vi "Control-CaseFlow.vi"(0 "Camera Device  IN":T1, 1 "Image Device IN":cluster{"Image":T5, "errorImage":errorcluster}, 2 "DAQ Device IN":T3={"DAQ Fs (S/s)"=10000.0, "task"="", "error"={"status"=FALSE, "code"=0, "source"=""}, "Min Value"=-10.0, "Max Value"=10.0}, 3 "Time Control Parameters":cluster{"# samples":u32, "tiempos (ms)":dbl}, 4 "Parametros Maximos":T6, 5 "detla Parametros":T6, 6 "Camara ON?":bool, 7 "Control Parameters":T4={"N Init Avg"=6, "N Avg Best"=3, "% Best to test"=0.95, "% Best to beat"=1.0}, 8 "Control?":bool=TRUE, 9 "Reset Control":bool, 10 "Ajuste?":bool=TRUE, 11 "Calibracion DAQ":T2) -> (13 "Status Text":string, 14 "Camera Device OUT":T1, 15 "Image Device OUT":cluster{"Image":T5, "errorImage":errorcluster}, 16 "DAQ Device OUT":T3={"DAQ Fs (S/s)"=0.0, "task"="", "error"={"status"=FALSE, "code"=0, "source"=""}, "Min Value"=-10.0, "Max Value"=10.0}, 17 "Contraste":dbl, 18 "Waveform":waveform(dbl), 19 "Señal de Control":dbl[](array[numeric]))   [LabVIEW 2010]
uses:
  <vilib>/vision/Image Controls.llb/IMAQ Image.ctl
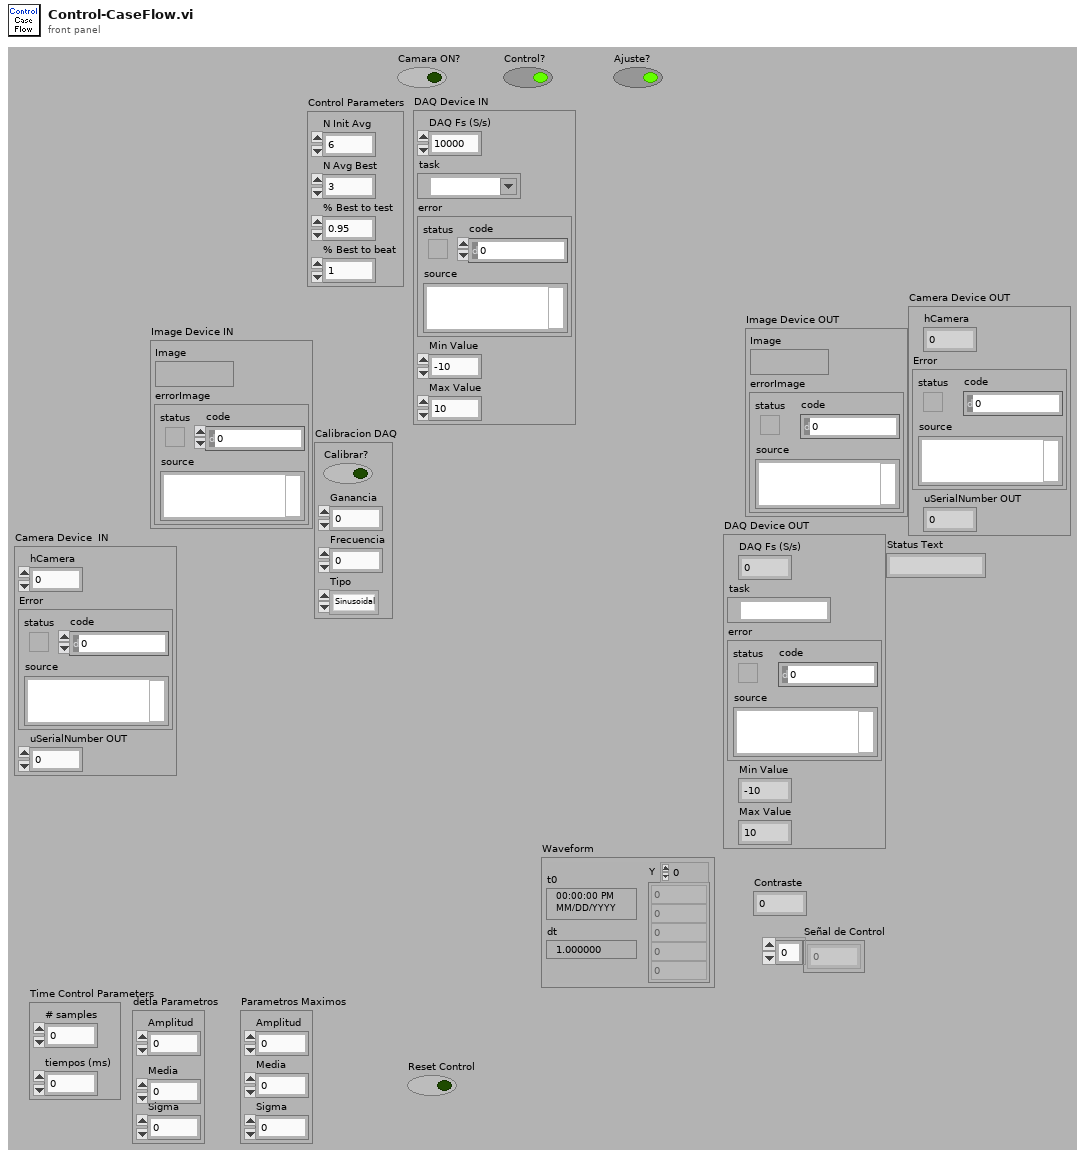
[diagram p1: front panel]
types:
  T1 = cluster{"hCamera":u32, "Error":errorcluster, "uSerialNumber OUT":u32}
  T2 = cluster{"Calibrar?":bool, "Ganancia":dbl, "Frecuencia":dbl, "Tipo":enum16{"Sinusoidal", "Triangular", "Cuadrada"}}
  T3 = cluster{"DAQ Fs (S/s)":dbl, "task":refnum<k21>, "error":errorcluster, "Min Value":dbl, "Max Value":dbl}
  T4 = cluster{"N Init Avg":u32, "N Avg Best":u32, "% Best to test":dbl, "% Best to beat":dbl}
  T5 = typedef "IMAQ Image.ctl" = refnum<image>
  T6 = cluster{"Amplitud":dbl, "Media":dbl, "Sigma":dbl}
  T7 = cluster{"DAQ Limits":cluster{"max":dbl, "min":dbl}, "Control Limits":cluster{"max":dbl, "min":dbl}}
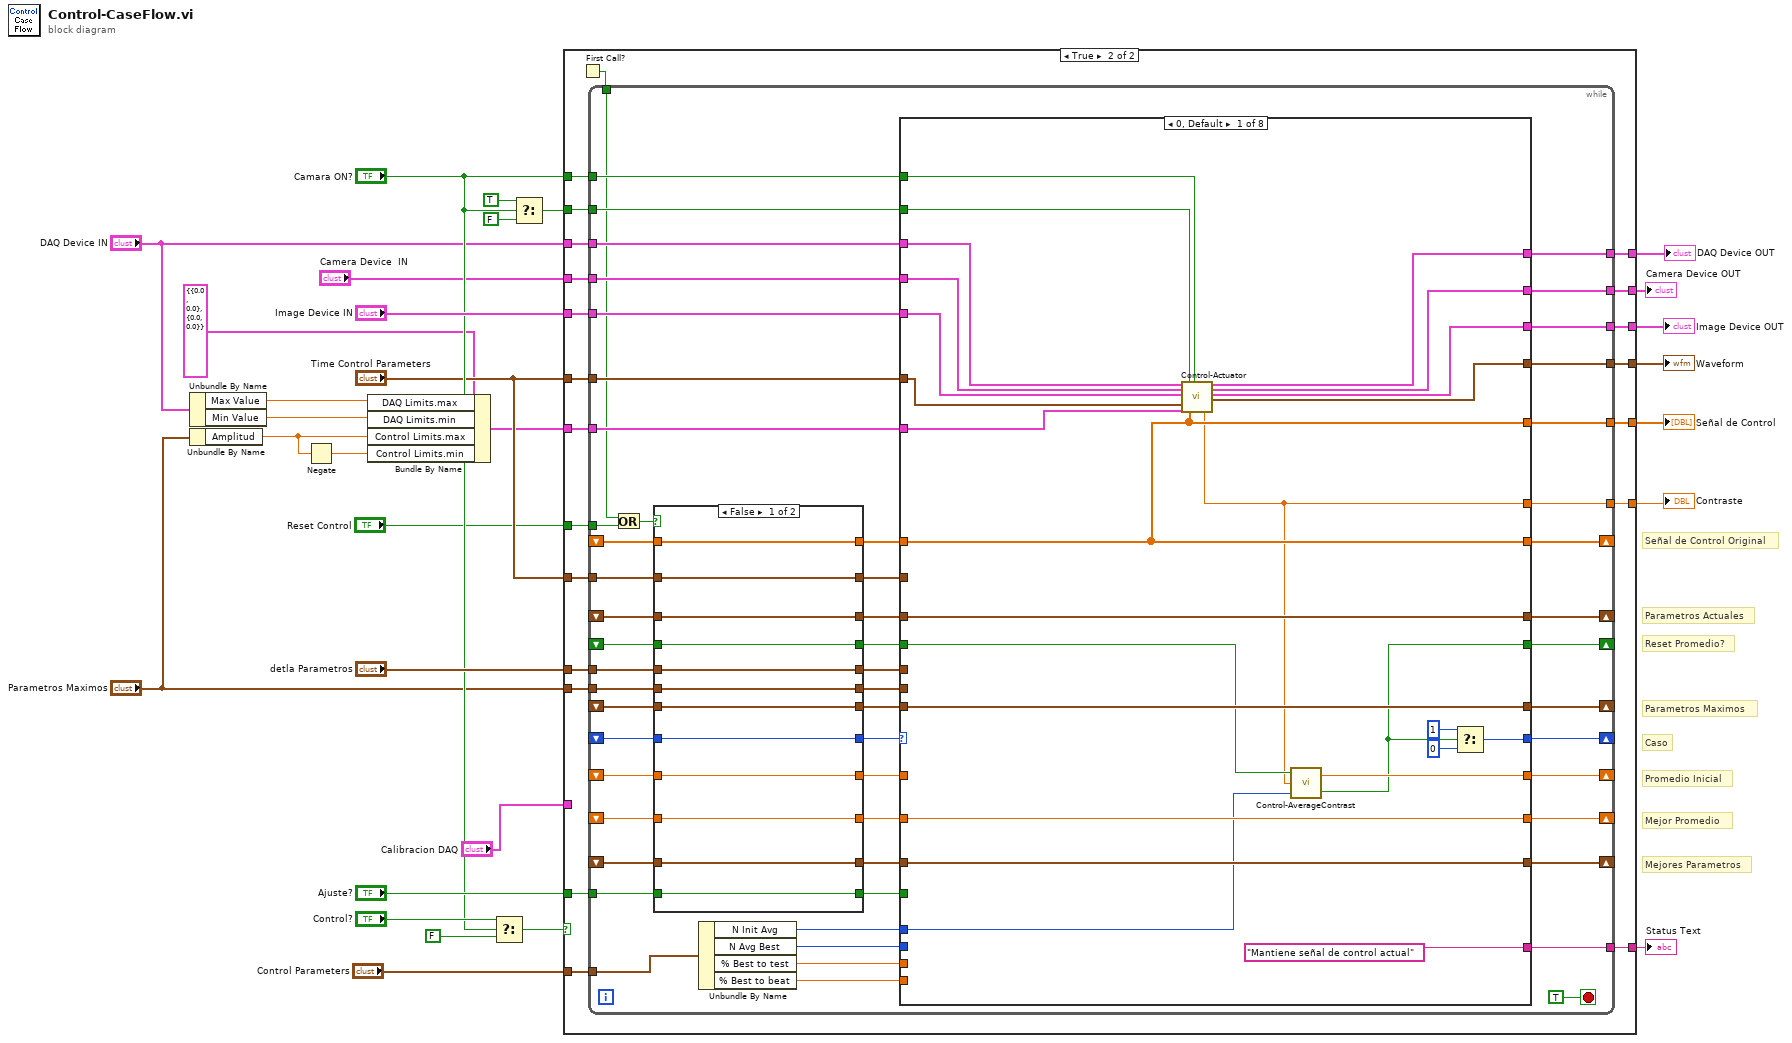
[diagram p0: block diagram]
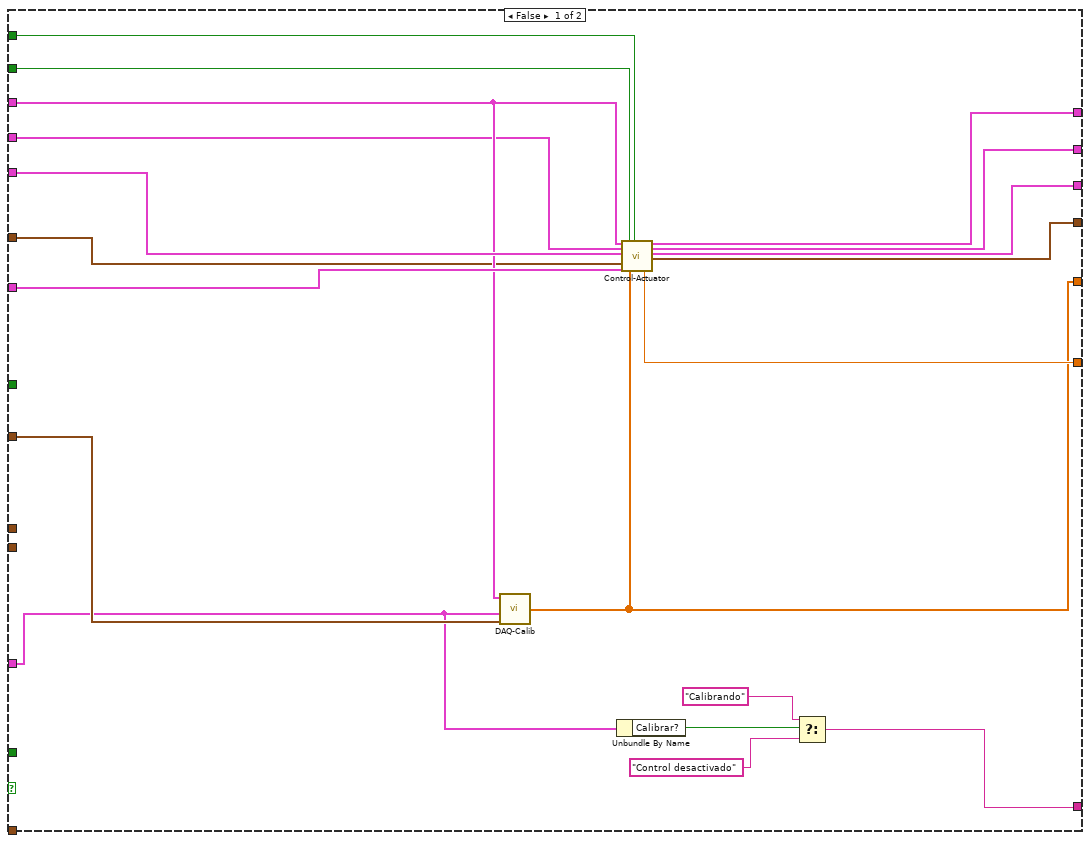
[diagram p2: hidden frame]
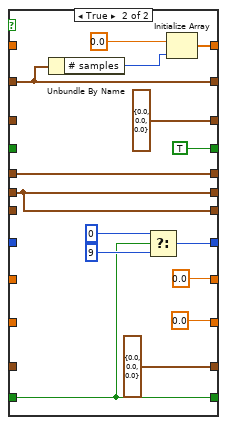
[diagram p3: hidden frame]
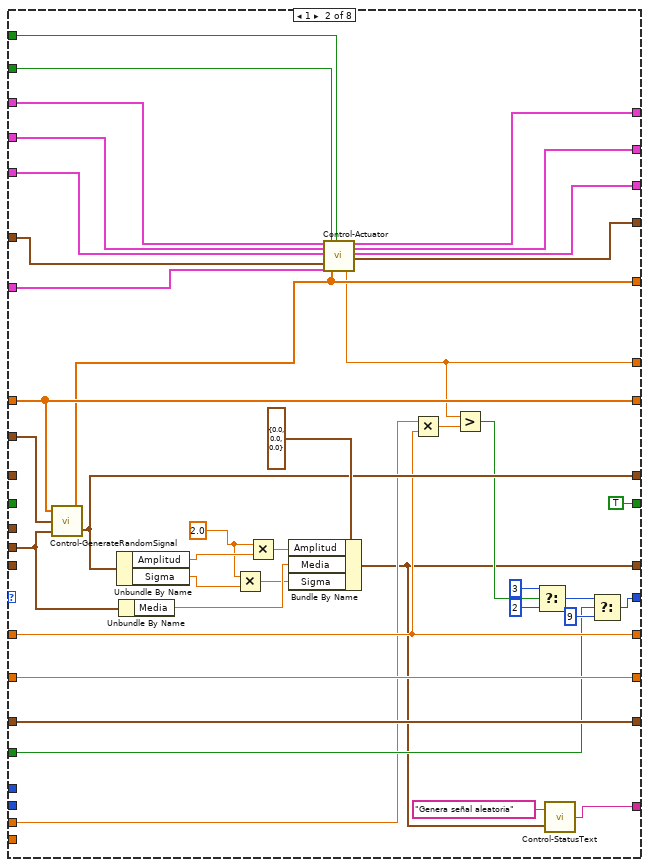
[diagram p4: hidden frame]
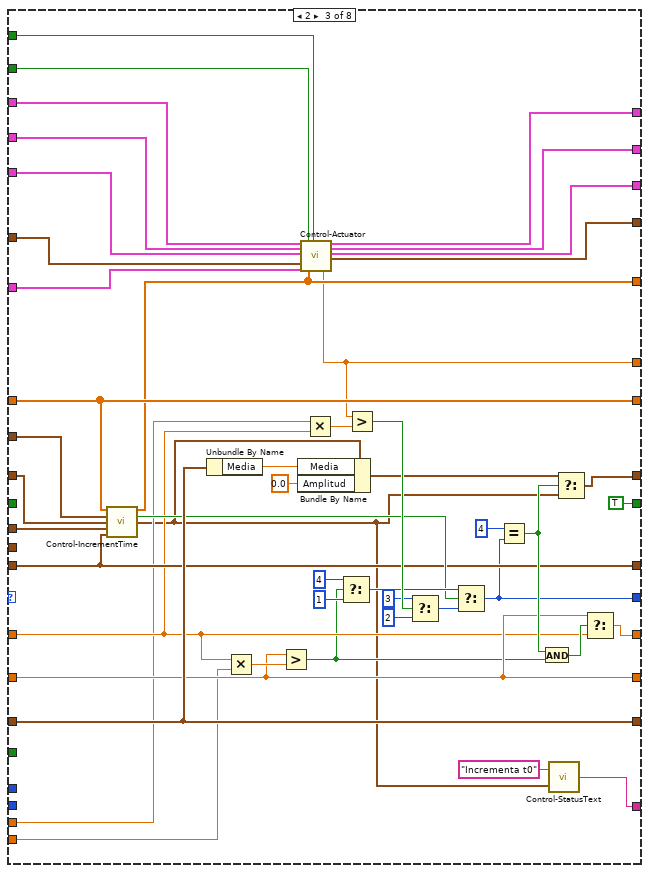
[diagram p5: hidden frame]
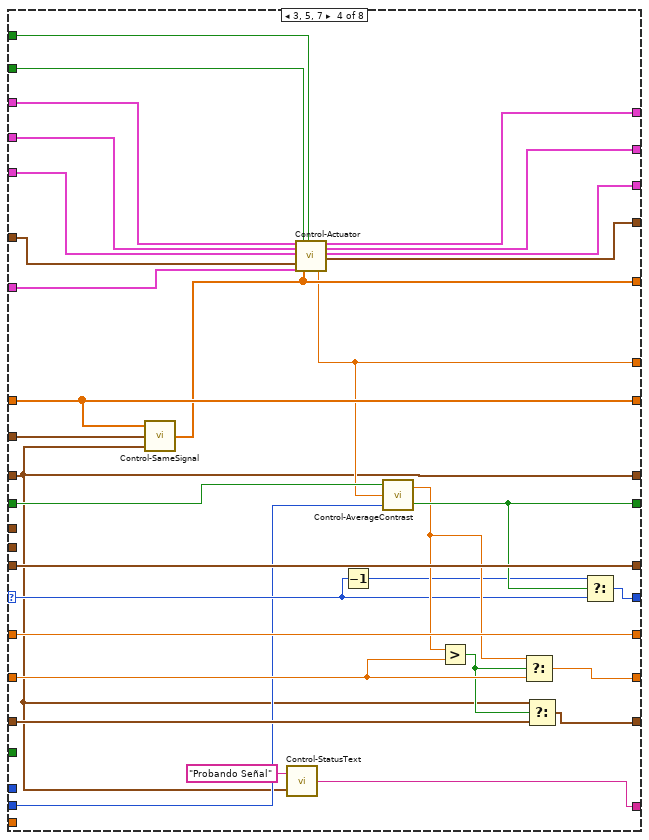
[diagram p6: hidden frame]
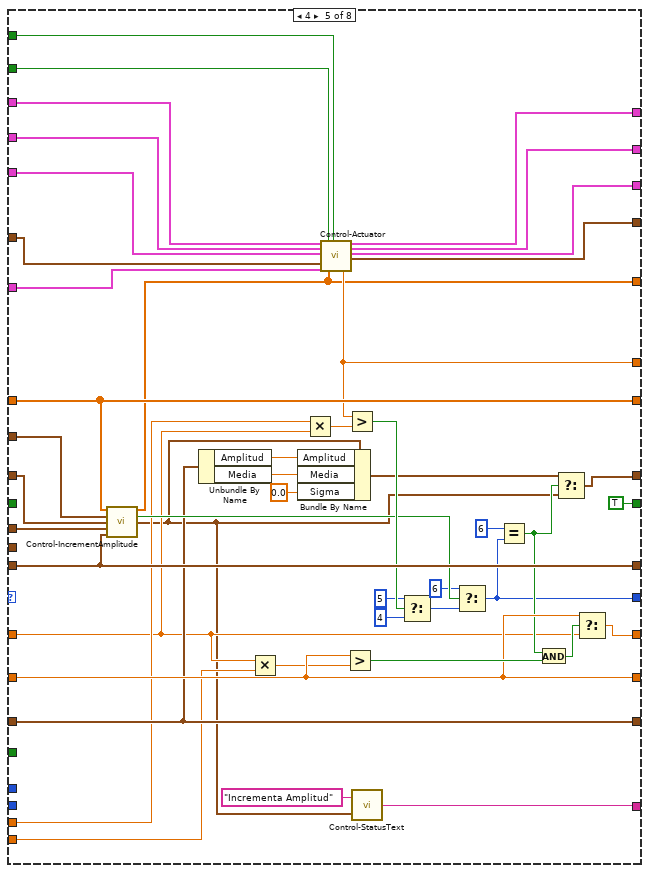
[diagram p7: hidden frame]
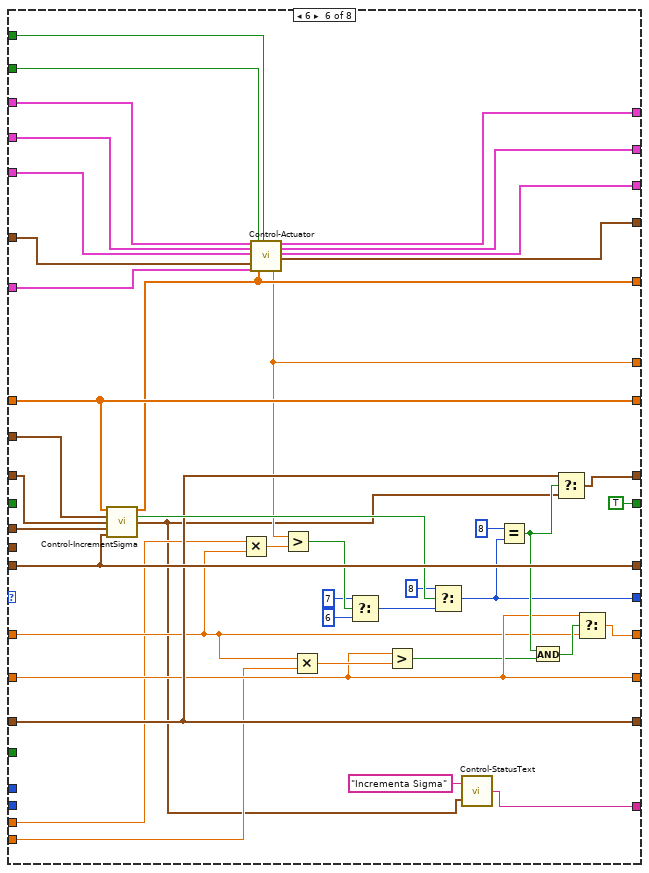
[diagram p8: hidden frame]
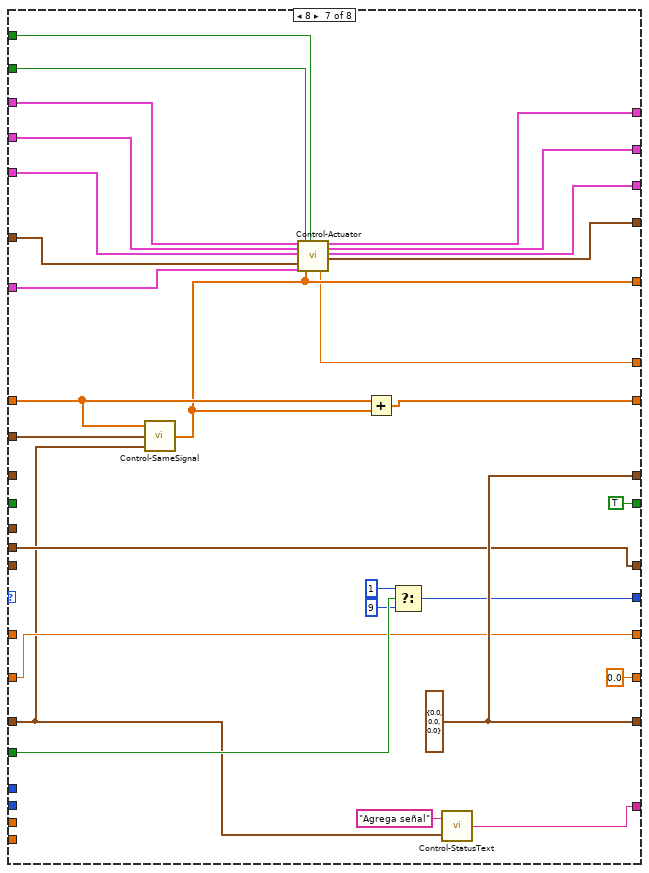
[diagram p9: hidden frame]
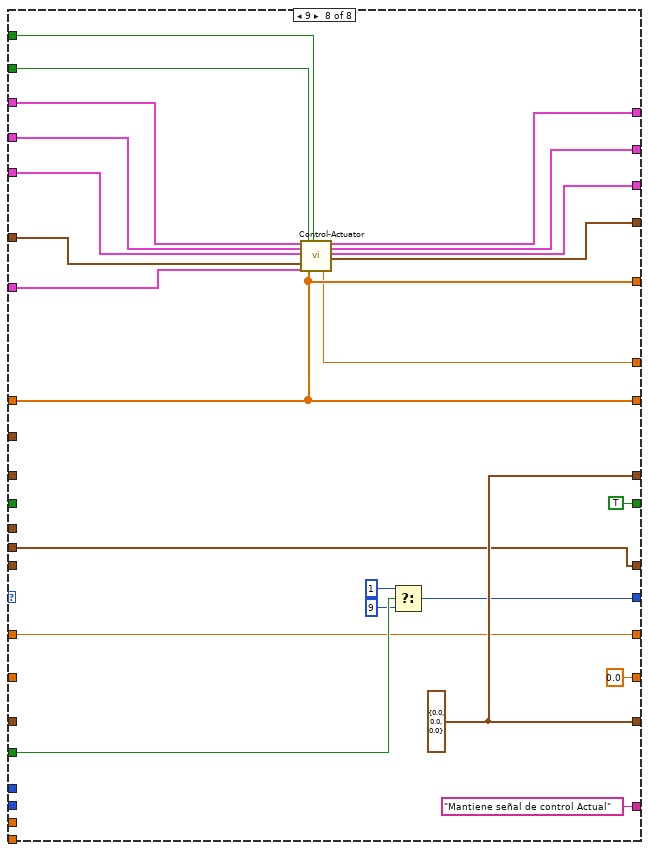
[diagram p10: hidden frame]
diagram:
  # "Reset Promedio?"
  # "Mejores Parametros"
  # "Mejor Promedio"
  # "Señal de Control Original"
  # "Parametros Actuales"
  # "Parametros Maximos"
  # "Caso"
  # "Promedio Inicial"
  n1 = Unbundle By Name("DAQ Device IN") -> ("Max Value"=w10:dbl, "Min Value"=w9:dbl)
  n2 = Unbundle By Name("Parametros Maximos") -> ("Amplitud"=w7:dbl)
  n3 = Negate(x=w7) -> (-x=w8:dbl)
  n4 = Bundle By Name(cluster=T7 {"DAQ Limits"={"max"=0.0, "min"=0.0}, "Control Limits"={"max"=0.0, "min"=0.0}} ("Limites"), "DAQ Limits.max"=w10, "DAQ Limits.min"=w9, "Control Limits.max"=w7, "Control Limits.min"=w8) -> (w11:T7)
  n5 = Select(t="Control?", s="Camara ON?", f=FALSE) -> (s? t:f=w20:bool)
  n6 = Select(t=TRUE, s="Camara ON?", f=FALSE) -> (s? t:f=w23:bool)
  n7 = case shown="True" w20 {
    tunnel: "Time Control Parameters" -> [w37 w70]
    tunnel: "detla Parametros" -> [_ w69]
    tunnel: "Parametros Maximos" -> [_ w68]
    tunnel: "Ajuste?" -> [_ w66]
    tunnel: [w39 w65] -> w28
    tunnel: [w49 w64] -> w27
    tunnel: w11 -> [w48 w63]
    tunnel: "Time Control Parameters" -> [w36 w62]
    tunnel: "Image Device IN" -> [w47 w61]
    tunnel: "Camera Device  IN" -> [w38 w60]
    tunnel: "DAQ Device IN" -> [w40 w59]
    tunnel: w23 -> [w46 w58]
    tunnel: "Camara ON?" -> [w45 w57]
    tunnel: [w44 w56] -> w25
    tunnel: [w43 w55] -> w24
    tunnel: [w42 w54] -> w2
    tunnel: [w41 w53] -> w13
    tunnel: "Reset Control" -> [_ w52]
    tunnel: "Control Parameters" -> [_ w51]
    tunnel: "Calibracion DAQ" -> [w32 _]
    tunnel: [w31 w50] -> w1
    frame False {
      n8 = call "DAQ-Calib.vi"("Time Control Parameters"=w37, "Calibracion DAQ"=w32, "DAQ Device IN"=w40) -> ("Calibration OUT"=w39:dbl[])  [unwired: 1 in]
      n9 = Unbundle By Name(w32) -> ("Calibrar?"=w35:bool)
      n10 = call "Control-Actuator.vi"("DAQ Device IN"=w40, "Camera Device  IN"=w38, "Image Device IN"=w47, "Time Control Parameters"=w36, "Limites"=w48, "DAQ?"=w46, "ControlSignal"=w39, "Streeam?"=w45) -> ("Contraste"=w49:dbl, "DAQ Device OUT"=w41:T3, "Camera Device OUT"=w42:T1, "Image Device OUT"=w43:cluster{"Image":T5, "errorImage":errorcluster}, "Waveform"=w44:waveform(dbl))  [unwired: 7 in]
      n11 = Select(t="Calibrando", s=w35, f="Control desactivado") -> (s? t:f=w31:string)
    }
    frame True {
      n12 = First Call?() -> (First Call?: T/F=w67:bool)
      n13 = while {
        shift-right: [w122] -> _
        shift-left: _ -> [w109]
        tunnel: w70 -> [w101]
        shift-right: [w125] -> _
        shift-left: _ -> [w117]
        shift-right: [w124] -> _
        shift-left: _ -> [w111]
        shift-right: [w123] -> _
        shift-left: _ -> [w115]
        shift-right: [w121] -> _
        shift-left: _ -> [w107]
        tunnel: w69 -> [w98]
        shift-right: [w120] -> _
        shift-left: _ -> [w105]
        shift-right: [w119] -> _
        shift-left: _ -> [w103]
        shift-right: [w118] -> _
        shift-left: _ -> [w113]
        tunnel: w66 -> [w100]
        tunnel: w68 -> [w99]
        tunnel: w67 -> [w79]
        tunnel: [w93] -> w65
        tunnel: [w92] -> w64
        tunnel: w63 -> [w91]
        tunnel: w62 -> [w90]
        tunnel: w61 -> [w89]
        tunnel: w60 -> [w88]
        tunnel: w59 -> [w87]
        tunnel: w58 -> [w86]
        tunnel: w57 -> [w85]
        tunnel: [w84] -> w56
        tunnel: [w83] -> w55
        tunnel: [w82] -> w54
        tunnel: [w81] -> w53
        tunnel: w52 -> [w77]
        tunnel: w51 -> [w76]
        tunnel: [w71] -> w50
        stop <- TRUE stop-if-true
        n14 = Or(x=w79, y=w77) -> (x .or. y?=w78:bool)
        n15 = case shown="False" w78 {
          tunnel: w117 -> [w137 _]
          tunnel: [w137 w152] -> w116
          tunnel: [w136 T6 {"Amplitud"=0.0, "Media"=0.0, "Sigma"=0.0} ("Parametros Iniciales")] -> w114
          tunnel: w115 -> [w136 _]
          tunnel: w113 -> [w135 _]
          tunnel: [w135 TRUE] -> w112
          tunnel: w111 -> [w134 _]
          tunnel: [w134 w141] -> w110
          tunnel: w109 -> [w133 _]
          tunnel: [w133 w142] -> w108
          tunnel: w107 -> [w132 _]
          tunnel: [w132 0.0 ("Contraste Promedio")] -> w106
          tunnel: w105 -> [w131 _]
          tunnel: [w131 0.0 ("Contraste Promedio")] -> w104
          tunnel: w103 -> [w130 _]
          tunnel: [w130 T6 {"Amplitud"=0.0, "Media"=0.0, "Sigma"=0.0} ("Parametros Maximos")] -> w102
          tunnel: w101 -> [w129 w138]
          tunnel: w99 -> [w127 w141]
          tunnel: w100 -> [w126 w139]
          tunnel: [w127 w141] -> w97
          tunnel: [w128 w140] -> w96
          tunnel: w98 -> [w128 w140]
          tunnel: [w126 w139] -> w95
          tunnel: [w129 w138] -> w94
          frame False {
          }
          frame True {
            n16 = Unbundle By Name(w138) -> ("# samples"=w150:u32)
            n17 = Select(t=u32 0, s=w139, f=u32 9) -> (s? t:f=w142:u32)
            n18 = Initialize Array(0.0 ("element"), w150) -> (w152:dbl[])
          }
        }
        n19 = Unbundle By Name(w76) -> ("N Init Avg"=w75:u32, "N Avg Best"=w74:u32, "% Best to test"=w73:dbl, "% Best to beat"=w72:dbl)
        n20 = case shown="0, Default" w108 {
          selector: w108 -> [_ _ _ w282 _ _ _ _]
          tunnel: w116 -> [w167 w216 w261 w295 w339 w381 w405 w426]
          tunnel: w94 -> [_ w217 w264 w296 w342 w384 w412 _]
          tunnel: w110 -> [w170 _ w245 w287 w338 w380 _ _]
          tunnel: [w167 w216 w261 w295 w339 w381 w404 w426] -> w125
          tunnel: [w170 w178 w245 w287 w338 w380 w401 w428] -> w124
          tunnel: [w171 w214 w251 w266 w328 w372 w410 w434] -> w123
          tunnel: [w177 w184 w229 w294 w307 w352 w402 w429] -> w122
          tunnel: [w172 w206 w255 w293 w333 w376 w403 w427] -> w121
          tunnel: w106 -> [_ w206 w224 w293 w300 w348 _ w427]
          tunnel: [w166 w185 w243 w280 w320 w367 w399 w425] -> w92
          tunnel: [w167 w200 w244 w281 w319 w368 w400 w426] -> w93
          tunnel: w114 -> [w171 _ w263 w266 w341 w383 _ _]
          tunnel: w96 -> [_ _ w262 _ w340 w382 _ _]
          tunnel: [w173 w209 w226 w292 w331 w350 0.0 ("Contraste Promedio") 0.0 ("Contraste Promedio")] -> w120
          tunnel: [w174 w208 w249 w290 w326 w369 w410 w434] -> w119
          tunnel: w102 -> [w174 w208 w249 w288 w326 w369 w385 _]
          tunnel: w104 -> [w173 w209 w226 w291 w331 w350 w403 _]
          tunnel: w112 -> [w168 _ _ w286 _ _ _ _]
          tunnel: [w169 TRUE ("Llego a N?") TRUE ("Llego a N?") w285 TRUE ("Llego a N?") TRUE ("Llego a N?") TRUE ("Llego a N?") TRUE ("Llego a N?")] -> w118
          tunnel: w95 -> [_ w186 _ _ _ _ w408 w432]
          tunnel: w97 -> [_ w201 _ _ _ _ w401 w428]
          tunnel: w91 -> [w165 w199 w242 w279 w304 w366 w398 w424]
          tunnel: w90 -> [w164 w198 w241 w278 w305 w363 w397 w423]
          tunnel: w89 -> [w163 w197 w240 w277 w318 w362 w396 w422]
          tunnel: w88 -> [w162 w196 w239 w276 w317 w361 w395 w421]
          tunnel: w87 -> [w161 w189 w238 w275 w306 w360 w394 w420]
          tunnel: w86 -> [w160 w195 w237 w274 w316 w364 w393 w419]
          tunnel: w85 -> [w159 w194 w236 w273 w315 w365 w392 w418]
          tunnel: [w158 w193 w235 w272 w314 w359 w391 w417] -> w84
          tunnel: [w157 w191 w234 w271 w313 w358 w390 w416] -> w83
          tunnel: [w156 w192 w233 w270 w312 w357 w389 w415] -> w82
          tunnel: [w155 w190 w232 w269 w311 w356 w388 w414] -> w81
          tunnel: w75 -> [w154 _ _ _ _ _ _ _]
          tunnel: w74 -> [_ _ _ w268 _ _ _ _]
          tunnel: w73 -> [_ w183 w222 _ w303 w347 _ _]
          tunnel: w72 -> [_ _ w225 _ w302 w349 _ _]
          tunnel: ["Mantiene señal de control actual" w180 w220 w267 w299 w345 w387 "Mantiene señal de control Actual"] -> w71
          frame 0, Default {
            n21 = call "Control-Actuator.vi"("DAQ Device IN"=w161, "Camera Device  IN"=w162, "Image Device IN"=w163, "Time Control Parameters"=w164, "Limites"=w165, "DAQ?"=w160, "ControlSignal"=w167, "Streeam?"=w159) -> ("Contraste"=w166:dbl, "DAQ Device OUT"=w155:T3, "Camera Device OUT"=w156:T1, "Image Device OUT"=w157:cluster{"Image":T5, "errorImage":errorcluster}, "Waveform"=w158:waveform(dbl))  [unwired: 7 in]
            n22 = call "Control-AverageContrast.vi"("N"=w154, "Contraste"=w166, "Reset"=w168) -> ("Llego a N?"=w169:bool, "Contraste Promedio"=w172:dbl)
            n23 = Select(t=u32 1, s=w169, f=u32 0) -> (s? t:f=w177:u32)
          }
          frame 1 {
            w210 = 2.0 ("x")
            n24 = call "Control-GenerateRandomSignal.vi"("Parametros Maximos"=w201, "Sound Parameters"=w217, "Señal de Control IN"=w216) -> ("Parametros Iniciales"=w214:T6, "Out"=w200:dbl[])
            n25 = Unbundle By Name(w214) -> ("Amplitud"=w213:dbl, "Sigma"=w211:dbl)
            n26 = Unbundle By Name(w201) -> ("Media"=w212:dbl)
            n27 = Multiply(x=w210, y=w211) -> (x*y=w181:dbl)
            n28 = Multiply(x=w210, y=w213) -> (x*y=w182:dbl)
            n29 = Bundle By Name(cluster=T6 {"Amplitud"=0.0, "Media"=0.0, "Sigma"=0.0} ("Parametros Iniciales"), "Amplitud"=w182, "Media"=w212, "Sigma"=w181) -> (w178:T6)
            n30 = call "Control-Actuator.vi"("DAQ Device IN"=w189, "Camera Device  IN"=w196, "Image Device IN"=w197, "Time Control Parameters"=w198, "Limites"=w199, "DAQ?"=w195, "ControlSignal"=w200, "Streeam?"=w194) -> ("Contraste"=w185:dbl, "DAQ Device OUT"=w190:T3, "Camera Device OUT"=w192:T1, "Image Device OUT"=w191:cluster{"Image":T5, "errorImage":errorcluster}, "Waveform"=w193:waveform(dbl))  [unwired: 7 in]
            n31 = Multiply(x=w183, y=w206) -> (x*y=w207:dbl)
            n32 = Greater?(x=w185, y=w207) -> (0:w205:bool)
            n33 = Select(t=u32 3, s=w205, f=u32 2) -> (s? t:f=w187:u32)
            n34 = call "Control-StatusText.vi"("Parametros Actuales"=w178, "string"="Genera señal aleatoria") -> ("String"=w180:string)
            n35 = Select(t=w187, s=w186, f=u32 9) -> (s? t:f=w184:u32)
          }
          frame 2 {
            n36 = call "Control-IncrementTime.vi"("Señal de Control IN"=w261, "Sound Parameters"=w264, "Parametros Actuales IN"=w263, "detla Parametros"=w262, "Parametros Maximos"=w245) -> ("Out"=w244:dbl[], "Tope?"=w247:bool, "Parametros Actuales OUT"=w219:T6)  [unwired: 8 in]
            n37 = Unbundle By Name(w249) -> ("Media"=w221:dbl)
            n38 = Multiply(x=w224, y=w225) -> (x*y=w227:dbl)
            n39 = Greater?(x=w226, y=w227) -> (0:w223:bool)
            n40 = Bundle By Name(cluster=w219, "Media"=w221, "Amplitud"=0.0) -> (w250:T6)
            n41 = call "Control-Actuator.vi"("DAQ Device IN"=w238, "Camera Device  IN"=w239, "Image Device IN"=w240, "Time Control Parameters"=w241, "Limites"=w242, "DAQ?"=w237, "ControlSignal"=w244, "Streeam?"=w236) -> ("Contraste"=w243:dbl, "DAQ Device OUT"=w232:T3, "Camera Device OUT"=w233:T1, "Image Device OUT"=w234:cluster{"Image":T5, "errorImage":errorcluster}, "Waveform"=w235:waveform(dbl))  [unwired: 7 in]
            n42 = Multiply(x=w222, y=w224) -> (x*y=w260:dbl)
            n43 = Select(t=u32 4, s=w223, f=u32 1) -> (s? t:f=w256:u32)
            n44 = Greater?(x=w243, y=w260) -> (0:w259:bool)
            n45 = Select(t=u32 3, s=w259, f=u32 2) -> (s? t:f=w228:u32)
            n46 = Select(t=w256, s=w247, f=w228) -> (s? t:f=w229:u32)
            n47 = Equal?(x=u32 4, y=w229) -> (x = y?=w246:bool)
            n48 = And(x=w246, y=w223) -> (x .and. y?=w254:bool)
            n49 = call "Control-StatusText.vi"("Parametros Actuales"=w219, "string"="Incrementa t0") -> ("String"=w220:string)
            n50 = Select(t=w250, s=w246, f=w219) -> (s? t:f=w251:T6)
            n51 = Select(t=w226, s=w254, f=w224) -> (s? t:f=w255:dbl)
          }
          frame 3, 5, 7 {
            n52 = call "Control-SameSignal.vi"("Parametros Actuales IN"=w266, "Sound Parameters"=w296, "Señal de Control IN"=w295) -> ("Out"=w281:dbl[])
            n53 = call "Control-StatusText.vi"("Parametros Actuales"=w266, "string"="Probando Señal") -> ("String"=w267:string)
            n54 = call "Control-Actuator.vi"("DAQ Device IN"=w275, "Camera Device  IN"=w276, "Image Device IN"=w277, "Time Control Parameters"=w278, "Limites"=w279, "DAQ?"=w274, "ControlSignal"=w281, "Streeam?"=w273) -> ("Contraste"=w280:dbl, "DAQ Device OUT"=w269:T3, "Camera Device OUT"=w270:T1, "Image Device OUT"=w271:cluster{"Image":T5, "errorImage":errorcluster}, "Waveform"=w272:waveform(dbl))  [unwired: 7 in]
            n55 = Decrement(x=w282) -> (x-1=w283:u32)
            n56 = call "Control-AverageContrast.vi"("N"=w268, "Contraste"=w280, "Reset"=w286) -> ("Llego a N?"=w285:bool, "Contraste Promedio"=w284:dbl)
            n57 = Greater?(x=w284, y=w291) -> (0:w289:bool)
            n58 = Select(t=w284, s=w289, f=w291) -> (s? t:f=w292:dbl)
            n59 = Select(t=w266, s=w289, f=w288) -> (s? t:f=w290:T6)
            n60 = Select(t=w283, s=w285, f=w282) -> (s? t:f=w294:u32)
          }
          frame 4 {
            n61 = call "Control-IncrementAmplitude.vi"("Señal de Control IN"=w339, "Sound Parameters"=w342, "Parametros Actuales IN"=w341, "detla Parametros"=w340, "Parametros Maximos"=w338) -> ("Out"=w319:dbl[], "Tope?"=w335:bool, "Parametros Actuales OUT"=w297:T6)  [unwired: 8 in]
            n62 = Unbundle By Name(w326) -> ("Amplitud"=w325:dbl, "Media"=w323:dbl)
            n63 = Multiply(x=w300, y=w302) -> (x*y=w301:dbl)
            n64 = Bundle By Name(cluster=w297, "Amplitud"=w325, "Media"=w323, "Sigma"=0.0 ("Amplitud")) -> (w327:T6)
            n65 = Multiply(x=w303, y=w300) -> (x*y=w337:dbl)
            n66 = call "Control-Actuator.vi"("DAQ Device IN"=w306, "Camera Device  IN"=w317, "Image Device IN"=w318, "Time Control Parameters"=w305, "Limites"=w304, "DAQ?"=w316, "ControlSignal"=w319, "Streeam?"=w315) -> ("Contraste"=w320:dbl, "DAQ Device OUT"=w311:T3, "Camera Device OUT"=w312:T1, "Image Device OUT"=w313:cluster{"Image":T5, "errorImage":errorcluster}, "Waveform"=w314:waveform(dbl))  [unwired: 7 in]
            n67 = Greater?(x=w331, y=w301) -> (0:w334:bool)
            n68 = Greater?(x=w320, y=w337) -> (0:w336:bool)
            n69 = call "Control-StatusText.vi"("Parametros Actuales"=w297, "string"="Incrementa Amplitud") -> ("String"=w299:string)
            n70 = Select(t=u32 5, s=w336, f=u32 4) -> (s? t:f=w308:u32)
            n71 = Select(t=u32 6, s=w335, f=w308) -> (s? t:f=w307:u32)
            n72 = Equal?(x=u32 6, y=w307) -> (x = y?=w321:bool)
            n73 = And(x=w321, y=w334) -> (x .and. y?=w332:bool)
            n74 = Select(t=w327, s=w321, f=w297) -> (s? t:f=w328:T6)
            n75 = Select(t=w331, s=w332, f=w300) -> (s? t:f=w333:dbl)
          }
          frame 6 {
            n76 = call "Control-IncrementSigma.vi"("Señal de Control IN"=w381, "Sound Parameters"=w384, "Parametros Actuales IN"=w383, "detla Parametros"=w382, "Parametros Maximos"=w380) -> ("Out"=w368:dbl[], "Tope?"=w377:bool, "Parametros Actuales OUT"=w344:T6)  [unwired: 8 in]
            n77 = Multiply(x=w347, y=w348) -> (x*y=w379:dbl)
            n78 = call "Control-Actuator.vi"("DAQ Device IN"=w360, "Camera Device  IN"=w361, "Image Device IN"=w362, "Time Control Parameters"=w363, "Limites"=w366, "DAQ?"=w364, "ControlSignal"=w368, "Streeam?"=w365) -> ("Contraste"=w367:dbl, "DAQ Device OUT"=w356:T3, "Camera Device OUT"=w357:T1, "Image Device OUT"=w358:cluster{"Image":T5, "errorImage":errorcluster}, "Waveform"=w359:waveform(dbl))  [unwired: 7 in]
            n79 = Greater?(x=w367, y=w379) -> (0:w378:bool)
            n80 = Multiply(x=w348, y=w349) -> (x*y=w351:dbl)
            n81 = Select(t=u32 7, s=w378, f=u32 6) -> (s? t:f=w353:u32)
            n82 = Greater?(x=w350, y=w351) -> (0:w346:bool)
            n83 = Select(t=u32 8, s=w377, f=w353) -> (s? t:f=w352:u32)
            n84 = call "Control-StatusText.vi"("Parametros Actuales"=w344, "string"="Incrementa Sigma") -> ("String"=w345:string)
            n85 = Equal?(x=u32 8, y=w352) -> (x = y?=w370:bool)
            n86 = And(x=w370, y=w346) -> (x .and. y?=w375:bool)
            n87 = Select(t=w369, s=w370, f=w344) -> (s? t:f=w372:T6)
            n88 = Select(t=w350, s=w375, f=w348) -> (s? t:f=w376:dbl)
          }
          frame 8 {
            w410 = T6 {"Amplitud"=0.0, "Media"=0.0, "Sigma"=0.0} ("Parametros Maximos")
            n89 = call "Control-SameSignal.vi"("Parametros Actuales IN"=w385, "Sound Parameters"=w412, "Señal de Control IN"=w405) -> ("Out"=w400:dbl[])
            n90 = call "Control-Actuator.vi"("DAQ Device IN"=w394, "Camera Device  IN"=w395, "Image Device IN"=w396, "Time Control Parameters"=w397, "Limites"=w398, "DAQ?"=w393, "ControlSignal"=w400, "Streeam?"=w392) -> ("Contraste"=w399:dbl, "DAQ Device OUT"=w388:T3, "Camera Device OUT"=w389:T1, "Image Device OUT"=w390:cluster{"Image":T5, "errorImage":errorcluster}, "Waveform"=w391:waveform(dbl))  [unwired: 7 in]
            n91 = Add(x=w405, y=w400) -> (x+y=w404:dbl[])
            n92 = Select(t=u32 1, s=w408, f=u32 9) -> (s? t:f=w402:u32)
            n93 = call "Control-StatusText.vi"("Parametros Actuales"=w385, "string"="Agrega señal") -> ("String"=w387:string)
          }
          frame 9 {
            w434 = T6 {"Amplitud"=0.0, "Media"=0.0, "Sigma"=0.0} ("Parametros Maximos")
            n94 = call "Control-Actuator.vi"("DAQ Device IN"=w420, "Camera Device  IN"=w421, "Image Device IN"=w422, "Time Control Parameters"=w423, "Limites"=w424, "DAQ?"=w419, "ControlSignal"=w426, "Streeam?"=w418) -> ("Contraste"=w425:dbl, "DAQ Device OUT"=w414:T3, "Camera Device OUT"=w415:T1, "Image Device OUT"=w416:cluster{"Image":T5, "errorImage":errorcluster}, "Waveform"=w417:waveform(dbl))  [unwired: 7 in]
            n95 = Select(t=u32 1, s=w432, f=u32 9) -> (s? t:f=w429:u32)
          }
        }
      }
    }
  }
  "Señal de Control" <- w28
  "Contraste" <- w27
  "Image Device OUT" <- w24
  "Waveform" <- w25
  "DAQ Device OUT" <- w13
  "Camera Device OUT" <- w2
  "Status Text" <- w1
